vi "BuildHeader.vi"() -> ()   [LabVIEW 2019]
panel:
  out "Result":string
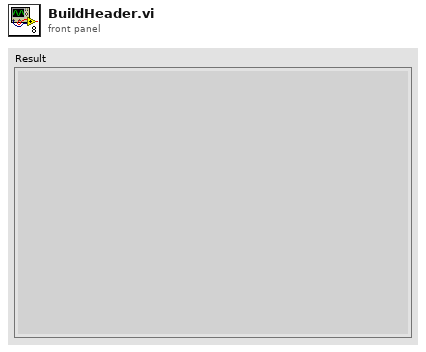
[diagram p1: front panel]
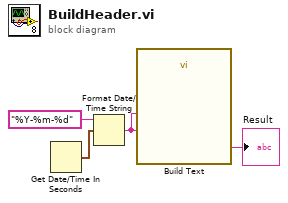
[diagram p0: block diagram]
diagram:
  n1 = Get Date/Time In Seconds() -> (seconds since 1Jan1904=w3:timestamp)
  n2 = Format Date/Time String(time format string (%c)="%Y-%m-%d", seconds (now)=w3) -> (date/time string=w1:string)  [unwired: 1 in]
  n3 = call "Build Text"("date"=w1, "date2"=w1) -> ("Result"=→"Result":string)  [unwired: 12 in, 1 out]
